vi "Auto_manual.vi"(1 "options":T1={"sp low"=0.0, "sp high"=100.0, "out low"=-100.0, "out high"=100.0, "hold (F)"=FALSE, "auto (T)"=TRUE, "pro. band (F)"=FALSE, "reverse acting (T)"=TRUE, "beta"=1.0, "linearity"=1.0, "dt (s)"=-1.0} {"dt (s)" format="%.2f"; "linearity" min=0.0 max=1.0 format="%.2f"; "sp low" format="%.2f"; "sp high" format="%.2f"; "out low" format="%.2f"; "out high" format="%.2f"; "beta" min=0.0 max=1.0 format="%.2f"}, 2 "manual control":dbl format="%.2f", 3 "auto control":dbl format="%.2f") -> (0 "output":dbl format="%.2f")   [LabVIEW 2017, in "NI_PID__prctrl compat.lvlib"]
doc: "This function handles auto-to-manual and manual-to-auto transfers."
uses:
  <vilib>/addons/control/pid/NI_PID__prctrl compat.lvlib
panel:
  # "SP & PV range:"
  # "Output range:"
  # "-1: default,using\nsystem clock"
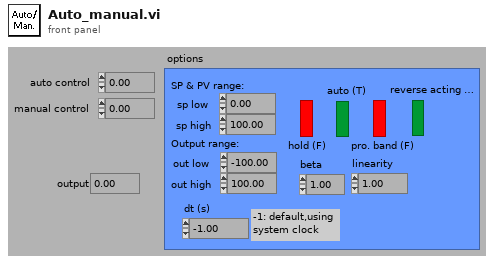
[diagram p1: front panel]
types:
  T1 = cluster{"sp low":dbl, "sp high":dbl, "out low":dbl, "out high":dbl, "hold (F)":bool, "auto (T)":bool, "pro. band (F)":bool, "reverse acting (T)":bool, "beta":dbl, "linearity":dbl, "dt (s)":dbl}
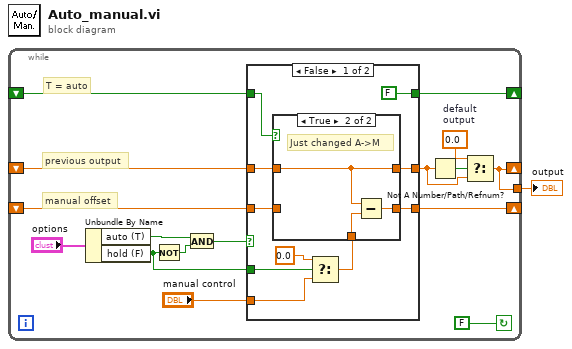
[diagram p0: block diagram]
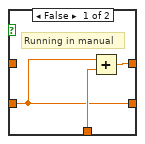
[diagram p2: hidden frame]
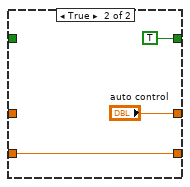
[diagram p3: hidden frame]
diagram:
  n1 = while {
    tunnel: [w4] -> w1
    shift-left: _ -> [w6]
    shift-right: [w4] -> _
    shift-left: _ -> [w9]
    shift-right: [w10] -> _
    shift-left: _ -> [w11]
    shift-right: [w12] -> _
    stop <- FALSE continue-if-true
    w5 = 0.0  # default output
    # "manual offset"
    # "previous output"
    # "T = auto"
    n2 = Unbundle By Name("options") -> ("auto (T)"=w16:bool, "hold (F)"=w13:bool)
    n3 = Not(x=w13) -> (.not. x?=w17:bool)
    n4 = And(x=w16, y=w17) -> (x .and. y?=w14:bool)
    n5 = case shown="False" w14 {
      tunnel: w13 -> [w21 _]
      tunnel: [FALSE TRUE] -> w12
      tunnel: w11 -> [w19 _]
      tunnel: [w26 "auto control"] -> w7
      tunnel: w6 -> [w25 _]
      tunnel: [w24 w34] -> w10
      tunnel: w9 -> [w23 w34]
      tunnel: "manual control" -> [w20 _]
      frame False {
        n6 = Select(t=0.0, s=w21, f=w20) -> (s? t:f=w18:dbl)
        n7 = case shown="True" w19 {
          tunnel: [w30 w33] -> w26
          tunnel: w25 -> [_ w33]
          tunnel: [w28 w32] -> w24
          tunnel: w23 -> [w28 _]
          tunnel: w18 -> [w29 w31]
          frame False {
            # "Running in manual"
            n8 = Add(x=w28, y=w29) -> (x+y=w30:dbl)
          }
          frame True {
            # "Just changed A->M"
            n9 = Subtract(x=w33, y=w31) -> (x-y=w32:dbl)
          }
        }
      }
      frame True {
      }
    }
    n10 = Not A Number/Path/Refnum?(number/path/refnum=w7) -> (NaN/Path/Refnum?=w3:bool)
    n11 = Select(t=w5, s=w3, f=w7) -> (s? t:f=w4:dbl)
  }
  "output" <- w1
